vi "Grab images from pco.edge or pco.pixelfly CL test1.vi"() -> ()   [LabVIEW 2015]
doc: "A short program to demonstrate the fundamentals of control and image acquision with the pco.camera series. The program records a sequence of images, with \"live\" updating, until the \"StopRecording\" button is pressed. Use ctrl-H for more help on the individual controls and indicators.\n\nCopyright 2004, 2010 The Cooke Corporation."
panel:
  out "cam_fps":dbl=20.079713544692744 caption="FPS" format="%.1g"
  out "bClose":bool
  in  "Quit":bool
  out "BufNr1":i16
  out "BufNr0":i16
  in  "bUseBuffer1":bool
  in  "bUseBuffer0":bool
  in  "ROIX1":u16=1 min=1
  in  "ROIY1":u16=1 min=1
  in  "ROIY0":u16=1 min=1
  in  "ROIX0":u16=1 min=1
  out "Bits/pixel":u16
  in  "Record":bool
  in  "DelayTimeBase":u16(ring)=2 items=["nanoseconds", "microseconds", "milliseconds"]
  in  "ExposureTimeBase":u16(ring)=2 items=["nanoseconds", "microseconds", "milliseconds"]
  in  "Exposure":u32=10
  in  "Delay":u32
  in  "Rate":i32(ring) items=["95333333", "286000000"]
  out "Image":u16[][](graph)
  in  "TriggerMode":u16(ring) items=["Auto", "Software", "External sequence start ", "External exposure control"]
  # "A short program to demonstrate the fundamentals of control and image acquision with the pco.camera series. The program records a sequence of images, with \"live\" updating, until the \"StopRecording\" button is pressed.  Use ctrl-H for more help on the individual controls and indicators."
  # "pco.labview"
  # "1) Setup camera:"
  # "2) Record  images:"
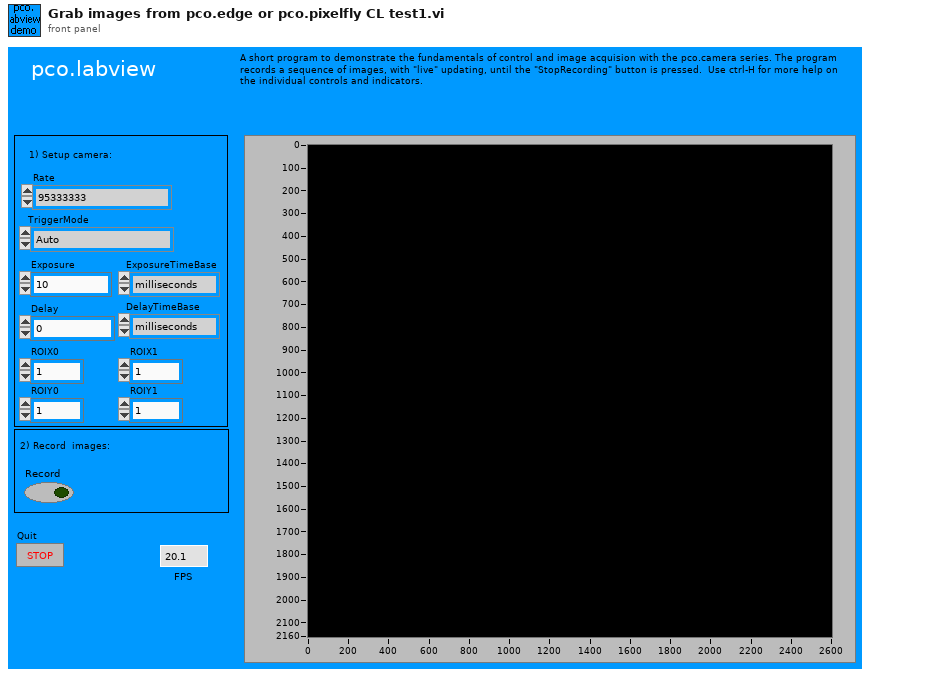
[diagram p1: front panel]
types:
  T1 = cluster{"SSize":u16, "CamType":u16, "CamsSubType":u16, "SerialNumber":u32, "HWVersion":u32, "FWVersion ":u32, "InterfaceType":u16, "HardwareVersions":cluster{"Board":u16, cluster{"string":string, "BatchNumber":u16, "MinorRevision":u8, "MajorRevision":u8, "Variant":u16}[]}, "FirmwareVersions":cluster{"DeviceNum":u16, cluster{"string":string, "MinorRevision":u8, "MajorRevision":u8, "Variant":u16}[]}}
  T2 = cluster{"Size":u16, "SensorTypeDESC":u16, "SensorSubtypeDESC":u16, "MaxHorizontalResStdDESC":u16, "MaxVerticalResStdDESC":u16, "MaxHorizontalResExtDESC":u16, "MaxVerticalResExtDESC":u16, "DynResDESC":u16, "MaxBinHorzDESC":u16, "BinHorzStepDESC":bool, "MaxBinVertDESC":u16, "BinVertStepDESC":bool, "ROIHorzStepDESC":u16, "ROIVertStepDESC":u16, "NumADCDESC":u16, "IRDESC":bool, "MinDelayDESC":u32, "MaxDelayDESC":u32, "MinDelayStepDESC":u32, "MinExpoDESC":u32, "MaxExpoDESC":u32, "MinExpoStepDESC":u32, "MinDelayIRDESC":u32, "MaxDelayIRDESC":u32, "MinExpoIRDESC":u32, "MaxExpoIRDESC":u32, "TimeTableDESC":bool, "DoubleImageDESC":bool, "MinCoolSetDESC":i16, "MaxCoolSetDESC":i16, "MDefaultCoolSetDESC":i16, "PowerDownModeDESC":bool, "OffsetRegDESC":bool, "ColorPattern":cluster{"UpperLeftColor":u8, "UpperRightColor":u8, "LowerLeftColor":u8, "LowerRightColor":u8}, "PatternTypeDESC":bool, "PixelRates":u32[], "CoversionFactors":u16[], "Reserved":u32[], "GeneralCapabilities":u32, "GeneralCapabilities 2":u32, "Min Size Hor":u16, "Min Size Vert":u16, "Ext Synch Freq":u32[], "Cooling Setpoints":i16[], "Soft ROI Hor Step":u16, "Soft ROI Vert Step":u16}
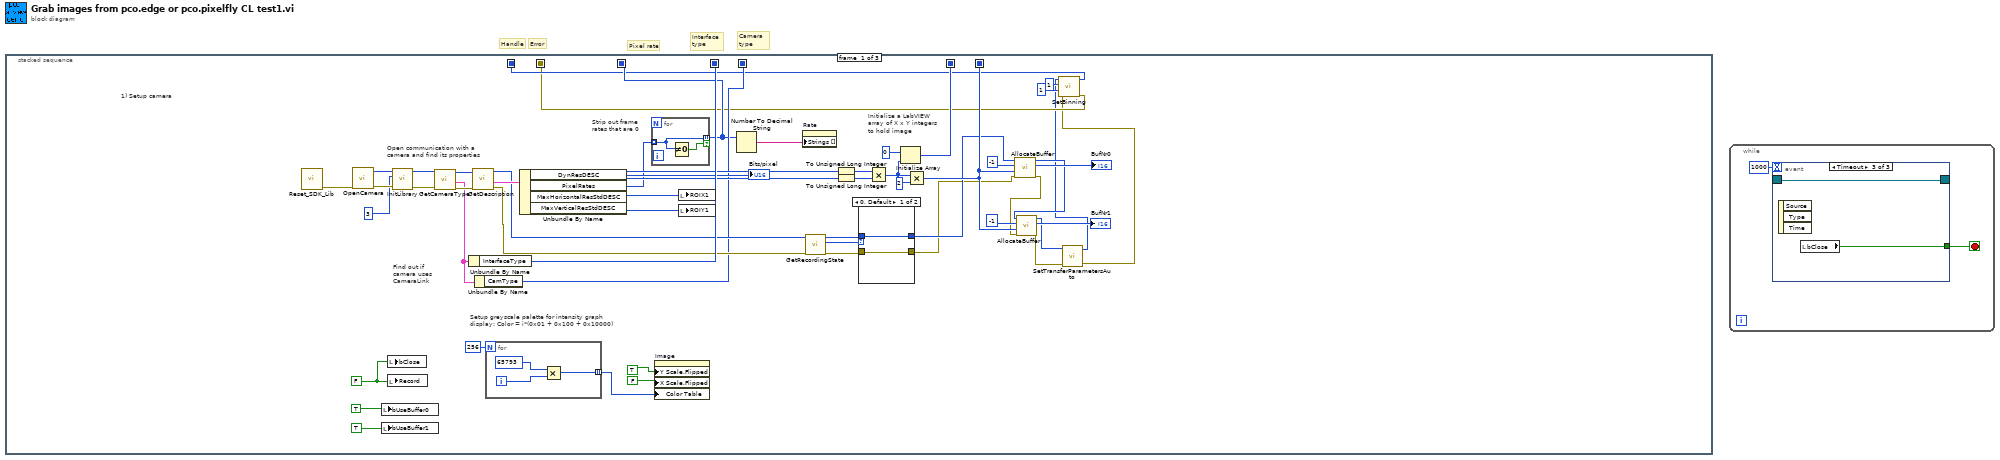
[diagram p0: block diagram]
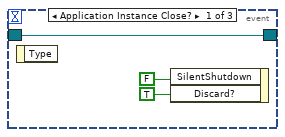
[diagram p2: hidden frame]
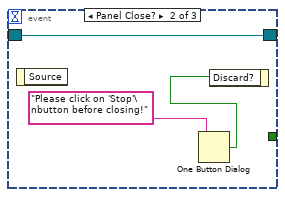
[diagram p3: hidden frame]
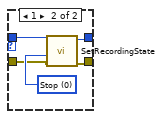
[diagram p4: hidden frame]
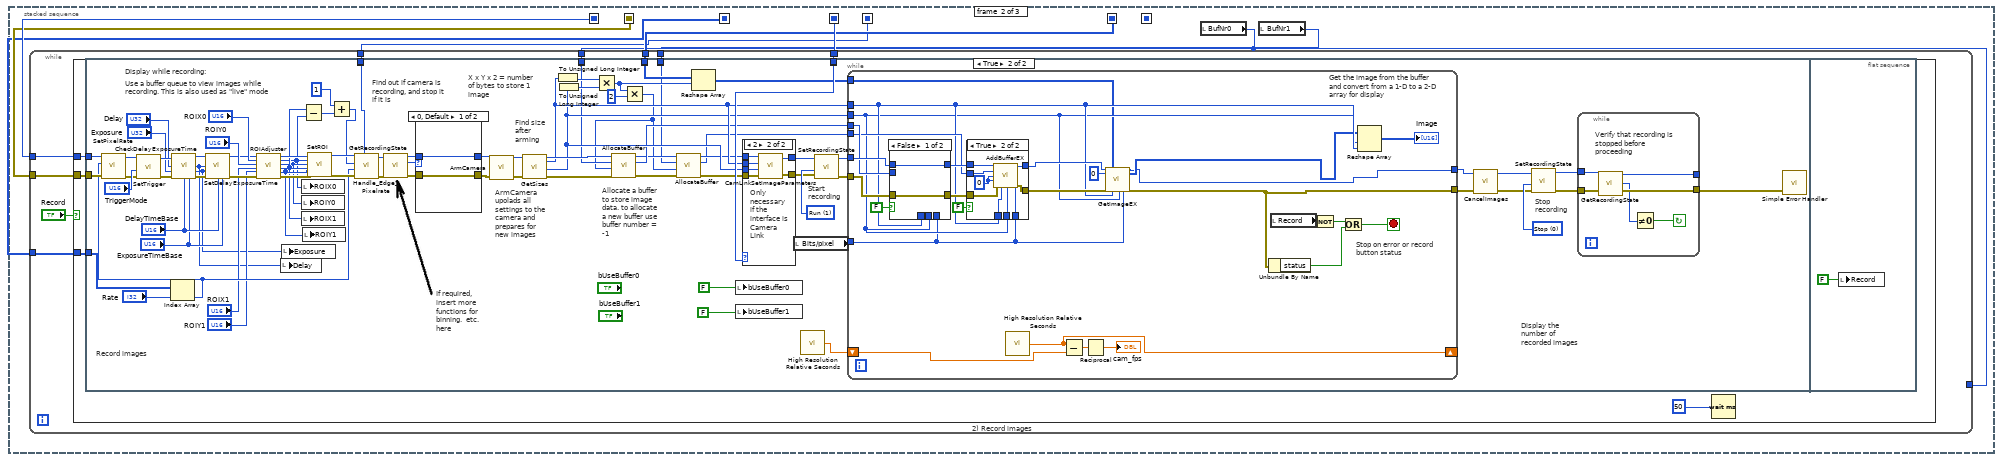
[diagram p5: hidden frame]
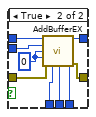
[diagram p7: hidden frame]
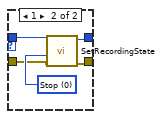
[diagram p10: hidden frame]
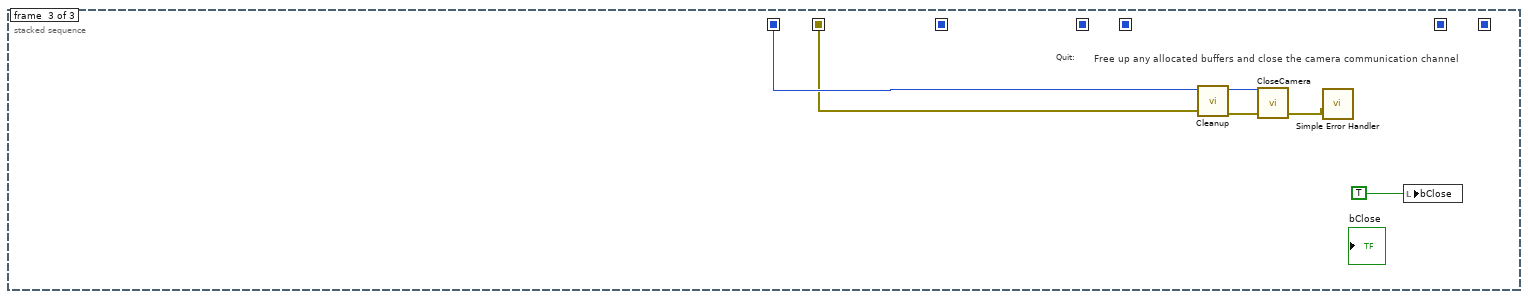
[diagram p11: hidden frame]
diagram:
  # "Camera type"
  # "Interface type"
  # "Error"
  # "Handle"
  # "Pixel rate"
  n1 = stacked-sequence {
    seq-local: [w47 _ _] -> [_ w70 _]
    seq-local: [w35 _ _] -> [_ _ _]
    seq-local: [w8 _ _] -> [_ w73 w247]
    seq-local: [w5 _ _] -> [_ w72 w246]
    seq-local: [w42 _ _] -> [_ w71 _]
    seq-local: [w9 _ _] -> [_ w67 _]
    seq-local: [w11 _ _] -> [_ w66 _]
    frame #0 {
      w29 = FALSE ("stop")
      # "Strip out frame rates that are 0"
      # "1) Setup camera"
      # "Find out if camera uses CameraLink"
      # "Setup greyscale palette for intensity graph display: Color = i*(0x01 + 0x100 + 0x10000)"
      # "Initialize a LabVIEW array of X x Y integers to hold image"
      # "Open communication with a camera and find its properties"
      n2 = call "Reset_SDK_Lib.vi"() -> ("ErrorOut"=w13:errorcluster)  [unwired: 11 in]
      n3 = call "OpenCamera.vi"("ErrorIn"=w13) -> ("ErrorOut"=w26:errorcluster, "Handle out"=w27:u64)  [unwired: 3 in, 2 out]
      n4 = local write "bUseBuffer0"(TRUE) -> ()
      n5 = local write "bUseBuffer1"(TRUE) -> ()
      n6 = local write "bClose"(w29) -> ()
      n7 = local write "Record"(w29) -> ()
      n8 = call "InitLibrary.vi"("error in (no error)"=w26, "InterfaceType"=u32 3, "ph"=w27) -> ("error out"=w25:errorcluster, "hout"=w24:u64)  [unwired: 7 in]
      n9 = call "GetCameraType.vi"("ph"=w24, "error in (no error)"=w25) -> ("hout"=w44:u64, "CameraType"=w12:T1, "error out"=w43:errorcluster)  [unwired: 1 in, 1 out]
      n10 = Unbundle By Name(w12) -> ("InterfaceType"=w42:u16)
      n11 = call "GetDescription.vi"("ErrorIn"=w43, "ph"=w44) -> ("ErrorOut"=w21:errorcluster, "Description"=w46:T2, "hout"=w20:u64)  [unwired: 2 in, 1 out]
      n12 = Unbundle By Name(w12) -> ("CamType"=w11:u16)
      n13 = for {
        N: 256 -> [_]
        tunnel: [w63] -> w50 mode=indexing
        i -> [w64]
        n14 = Multiply(x=65793, y=w64) -> (x*y=w63:i32)
      }
      n15 = Unbundle By Name(w46) -> ("DynResDESC"=→"Bits/pixel":u16, "PixelRates"=w10:u32[], "MaxHorizontalResStdDESC"=w40:u16, "MaxVerticalResStdDESC"=w39:u16)
      n16 = for {
        tunnel: w10 -> [w54] mode=indexing
        tunnel: [w54] -> w9 mode=indexing if=w55
        n17 = Not Equal To 0?(x=w54) -> (x != 0?=w55:bool)
      }
      n18 = property on="Image" class="IntGraph (strict)"("Y Scale.Flipped"=TRUE, "X Scale.Flipped"=FALSE, "Color Table"=w50) -> ()  [unwired: 2 in, 2 out]
      n19 = local write "ROIX1"(w40) -> ()
      n20 = local write "ROIY1"(w39) -> ()
      n21 = Number To Decimal String(number=w9) -> (decimal integer string=w28:string[])  [unwired: 1 in]
      n22 = property on="Rate" class="Ring (strict)"("Strings []"=w28) -> ()  [unwired: 2 in, 2 out]
      n23 = call "GetRecordingState.vi"("ErrorIn"=w21, "ph"=w20) -> ("ErrorOut"=w18:errorcluster, "Error"=w14:i32, "hout"=w19:u64)  [unwired: 2 in, 1 out]
      n24 = To Unsigned Long Integer(number=w40) -> (unsigned 32bit integer=w37:u32)
      n25 = To Unsigned Long Integer(number=w39) -> (unsigned 32bit integer=w36:u32)
      n26 = case shown="0, Default" w14 {
        tunnel: w19 -> [w57 w61]
        tunnel: w18 -> [w56 w60]
        tunnel: [w57 w59] -> w17
        tunnel: [w56 w58] -> w15
        frame 0, Default {
        }
        frame 1 {
          w62 = u16 0 items=["Stop", "Run"] ("RecordingState")
          n27 = call "SetRecordingState.vi"("ErrorIn"=w60, "RecordingState"=w62, "ph"=w61) -> ("ErrorOut"=w58:errorcluster, "hout"=w59:u64)  [unwired: 2 in, 1 out]
        }
      }
      n28 = Multiply(x=w37, y=w36) -> (x*y=w48:u32)
      n29 = Initialize Array(u16 0 ("Element Data"), w48) -> (w47:u16[])
      n30 = Multiply(x=w48, y=u32 2) -> (x*y=w35:u32)
      n31 = call "AllocateBuffer.vi"("error in (no error)"=w15, "Size"=w35, "BufNr"=i16 -1, "ph"=w17) -> ("error out"=w22:errorcluster, "BufNrOut"=→"BufNr0":i16, "hout"=w16:u64)  [unwired: 2 in, 3 out]
      n32 = call "AllocateBuffer.vi"("error in (no error)"=w22, "Size"=w35, "BufNr"=i16 -1, "ph"=w16) -> ("error out"=w2:errorcluster, "BufNrOut"=→"BufNr1":i16, "hout"=w4:u64)  [unwired: 2 in, 3 out]
      n33 = call "SetTransferParametersAuto.vi"("error in (no error)"=w2, "ph"=w4) -> ("error out"=w1:errorcluster, "hout"=w3:u64)  [unwired: 2 in, 1 out]
      n34 = call "SetBinning.vi"("error in (no error)"=w1, "BinVert"=u16 1, "BinHorz"=u16 1, "ph"=w3) -> ("error out"=w5:errorcluster, "hout"=w8:u64)  [unwired: 3 in, 1 out]
    }
    frame #1 {
      n35 = local read "BufNr0"() -> (w69:i16)
      n36 = local read "BufNr1"() -> (w68:i16)
      n37 = while {
        tunnel: w69 -> [_]
        tunnel: w69 -> [w79]
        tunnel: w70 -> [w81]
        tunnel: w71 -> [w82]
        tunnel: w72 -> [w80]
        tunnel: w73 -> [w77]
        tunnel: w68 -> [w78]
        tunnel: w67 -> [w75]
        tunnel: w66 -> [w74]
        stop <- "Quit" stop-if-true
        n38 = case "2) Record images" shown="True" "Record" {
          tunnel: w77 -> [_ w92]
          tunnel: w80 -> [_ w91]
          tunnel: w82 -> [_ w90]
          tunnel: w81 -> [_ w89]
          tunnel: w79 -> [_ w88]
          tunnel: w78 -> [_ w87]
          tunnel: w75 -> [_ w86]
          tunnel: w74 -> [_ w85]
          frame False {
          }
          frame True {
            n39 = flat-sequence {
              tunnel: w92 -> [w158]
              tunnel: w91 -> [w157]
              tunnel: w90 -> [w155]
              tunnel: w89 -> [w153]
              tunnel: w88 -> [w144]
              tunnel: w87 -> [w138]
              tunnel: w86 -> [w125]
              tunnel: w85 -> [w116]
              frame #0 {
                w171 = u16 1 items=["Stop", "Run"] ("RecordingState")
                w174 = u16 0 items=["Stop", "Run"] ("RecordingState")
                # "Display the number of recorded images"
                # "Record images"
                # "Start recording"
                # "Allocate a buffer to store image data. to allocate a new buffer use buffer number = -1"
                # "Find size after arming"
                # "ArmCamera upolads all settings to the camera and prepares for new images"
                # "Find out if camera is recording, and stop it if it is"
                # "If required, insert more functions for binning.  etc. here"
                # "X x Y x 2 = number of bytes to store 1 image"
                # "Stop recording"
                # "Use a buffer queue to view images while recording. This is also used as \"live\" mode"
                # "Display while recording:"
                n40 = Index Array(array=w125, index="Rate") -> (element=w120:u32)
                n41 = call "SetPixelRate.vi"("error in (no error)"=w157, "PixelRate"=w120, "ph"=w158) -> ("error out"=w127:errorcluster, "hout"=w128:u64)  [unwired: 2 in, 1 out]
                n42 = call "SetTrigger.vi"("error in (no error)"=w127, "TriggerMode"="TriggerMode", "ph"=w128) -> ("error out"=w101:errorcluster, "hout"=w103:u64)  [unwired: 2 in, 1 out]
                n43 = call "CheckDelayExposureTime.vi"("ph"=w103, "Delay"="Delay", "Exposure"="Exposure", "error in (no error)"=w101, "DelayTimeBase"="DelayTimeBase", "ExposureTimeBase"="ExposureTimeBase") -> ("hout"=w102:u64, "Delay Out"=w95:u32, "Exposure Out"=w94:u32, "error out"=w96:errorcluster)  [unwired: 4 in, 2 out]
                n44 = call "SetDelayExposureTime.vi"("ph"=w102, "Delay"=w95, "Exposure"=w94, "error in (no error)"=w96, "DelayTimeBase"="DelayTimeBase", "ExposureTimeBase"="ExposureTimeBase") -> ("hout"=w109:u64, "error out"=w115:errorcluster)  [unwired: 7 in, 1 out]
                n45 = call "ROIAdjuster.vi"("HandleIn"=w109, "ROIXmin"="ROIX0", "ROIYmin"="ROIY0", "ROIXmax"="ROIX1", "ROIYmax"="ROIY1", "ErrorIn"=w115) -> ("hout"=w108:u64, "ROIX0Mod"=w104:u16, "ROIY0Mod"=w105:u16, "ROIX1Mod"=w106:u16, "ROIY1Mod"=w107:u16, "ErrorOut"=w114:errorcluster)  [unwired: 7 in, 1 out]
                n46 = local write "Delay"(w95) -> ()
                n47 = local write "Exposure"(w94) -> ()
                n48 = Subtract(x=w106, y=w104) -> (x-y=w119:u16)
                n49 = local write "ROIX0"(w104) -> ()
                n50 = local write "ROIY0"(w105) -> ()
                n51 = local write "ROIX1"(w106) -> ()
                n52 = local write "ROIY1"(w107) -> ()
                n53 = call "SetROI.vi"("ph"=w108, "ROIX0"=w104, "ROIY0"=w105, "ROIX1"=w106, "ROIY1"=w107, "error in (no error)"=w114) -> ("hout"=w121:u64, "error out"=w122:errorcluster)  [unwired: 12 in]
                n54 = Add(x=1, y=w119) -> (x+y=w117:i32)
                n55 = call "Handle_Edge_Pixelrate.vi"("Cameratype"=w116, "error in (no error)"=w122, "PixelRate"=w120, "X-Resolution"=w117, "ph"=w121) -> ("error out"=w123:errorcluster, "hout"=w124:u64)  [unwired: 5 in]
                n56 = call "GetRecordingState.vi"("ErrorIn"=w123, "ph"=w124) -> ("ErrorOut"=w168:errorcluster, "RecordingState"=w170:u16, "hout"=w169:u64)  [unwired: 2 in, 1 out]
                n57 = case shown="0, Default" w170 {
                  tunnel: w169 -> [w239 w243]
                  tunnel: w168 -> [w238 w242]
                  tunnel: [w239 w241] -> w167
                  tunnel: [w238 w240] -> w166
                  frame 0, Default {
                  }
                  frame 1 {
                    w244 = u16 0 items=["Stop", "Run"] ("RecordingState")
                    n58 = call "SetRecordingState.vi"("ErrorIn"=w242, "RecordingState"=w244, "ph"=w243) -> ("ErrorOut"=w240:errorcluster, "hout"=w241:u64)  [unwired: 2 in, 1 out]
                  }
                }
                n59 = call "ArmCamera.vi"("error in (no error)"=w166, "ph"=w167) -> ("error out"=w164:errorcluster, "hout"=w165:u64)  [unwired: 1 in, 1 out]
                n60 = call "GetSizes.vi"("ph"=w165, "ErrorIn"=w164) -> ("hout"=w161:u64, "XResAct"=w151:u16, "YResAct"=w150:u16, "ErrorOut"=w163:errorcluster)  [unwired: 11 in, 3 out]
                n61 = To Unsigned Long Integer(number=w151) -> (unsigned 32bit integer=w145:u32)
                n62 = To Unsigned Long Integer(number=w150) -> (unsigned 32bit integer=w146:u32)
                n63 = Multiply(x=w145, y=w146) -> (x*y=w147:u32)
                n64 = Multiply(x=w147, y=u32 2) -> (x*y=w139:u32)
                n65 = call "AllocateBuffer.vi"("error in (no error)"=w163, "Size"=w139, "BufNr"=w144, "ph"=w161) -> ("error out"=w143:errorcluster, "BufNrOut"=w148:i16, "hout"=w141:u64)  [unwired: 2 in, 3 out]
                n66 = call "AllocateBuffer.vi"("error in (no error)"=w143, "Size"=w139, "BufNr"=w138, "ph"=w141) -> ("error out"=w142:errorcluster, "BufNrOut"=w137:i16, "hout"=w140:u64)  [unwired: 2 in, 3 out]
                n67 = Reshape Array(w153, w147) -> (w152:u16[])
                n68 = local write "bUseBuffer0"(FALSE) -> ()
                n69 = local write "bUseBuffer1"(FALSE) -> ()
                n70 = case shown="2" w155 {
                  tunnel: w142 -> [w230 w237]
                  tunnel: [w230 w236] -> w160
                  tunnel: w140 -> [w231 w235]
                  tunnel: [w231 w234] -> w159
                  tunnel: w150 -> [_ w233]
                  tunnel: w151 -> [_ w232]
                  frame 0, Default {
                  }
                  frame 2 {
                    # "Only necessary if the interface is Camera Link"
                    n71 = call "CamLinkSetImageParameters.vi"("error in (no error)"=w237, "YRes"=w233, "XRes"=w232, "ph"=w235) -> ("error out"=w236:errorcluster, "hout"=w234:u64)  [unwired: 1 out]
                  }
                }
                n72 = local read "Bits/pixel"() -> (w132:u16)
                n73 = call <vilib>:"High Resolution Relative Seconds.vi"() -> ("relative seconds"=w93:dbl)
                n74 = call "SetRecordingState.vi"("ErrorIn"=w160, "RecordingState"=w171, "ph"=w159) -> ("ErrorOut"=w156:errorcluster, "hout"=w154:u64)  [unwired: 2 in, 1 out]
                n75 = while {
                  tunnel: w148 -> [w195]
                  tunnel: w152 -> [w177]
                  tunnel: w154 -> [w200]
                  tunnel: w150 -> [w182]
                  tunnel: w151 -> [w183]
                  tunnel: w156 -> [w198]
                  tunnel: [w179] -> w131
                  tunnel: [w178] -> w130
                  tunnel: w137 -> [w194]
                  tunnel: w132 -> [w181]
                  shift-right: [w187] -> _
                  shift-left: w93 -> [w188]
                  stop <- w191 stop-if-true
                  # "Stop on error or record button status"
                  # "Get the image from the buffer and convert from a 1-D to a 2-D array for display"
                  n76 = case shown="False" FALSE {
                    tunnel: [w203 w212] -> w197
                    tunnel: [w202 w211] -> w199
                    tunnel: w195 -> [_ w210]
                    tunnel: w200 -> [w202 w209]
                    tunnel: w181 -> [_ w207]
                    tunnel: w183 -> [_ w206]
                    tunnel: w182 -> [_ w205]
                    tunnel: w198 -> [w203 w204]
                    frame False {
                    }
                    frame True {
                      w208 = i16 0
                      n77 = call "AddBufferEX.vi"("ph"=w209, "BuffNr"=w210, "1stImage"=w208, "LastImage"=w208, "error in (no error)"=w204, "XRes"=w206, "YRes"=w205, "BitPerPixel"=w207) -> ("hout"=w211:u64, "error out"=w212:errorcluster)  [unwired: 5 in, 1 out]
                    }
                  }
                  n78 = case shown="True" FALSE {
                    tunnel: [w213 w223] -> w186
                    tunnel: [w214 w222] -> w184
                    tunnel: w194 -> [_ w221]
                    tunnel: w199 -> [w214 w220]
                    tunnel: w181 -> [_ w218]
                    tunnel: w183 -> [_ w217]
                    tunnel: w182 -> [_ w216]
                    tunnel: w197 -> [w213 w215]
                    frame False {
                    }
                    frame True {
                      w219 = i16 0
                      n79 = call "AddBufferEX.vi"("ph"=w220, "BuffNr"=w221, "1stImage"=w219, "LastImage"=w219, "error in (no error)"=w215, "XRes"=w217, "YRes"=w216, "BitPerPixel"=w218) -> ("hout"=w222:u64, "error out"=w223:errorcluster)  [unwired: 5 in, 1 out]
                    }
                  }
                  n80 = call <vilib>:"High Resolution Relative Seconds.vi"() -> ("relative seconds"=w187:dbl)
                  n81 = Subtract(x=w187, y=w188) -> (x-y=w190:dbl)
                  n82 = Reciprocal(x=w190) -> (1/x=→"cam_fps":dbl)
                  n83 = call "GetImageEX.vi"("ph"=w184, "BuffNr"=i16 0, "error in (no error)"=w186, "BuffIn"=w177, "xRes"=w183, "yRes"=w182, "BitPerPixel"=w181) -> ("hout"=w179:u64, "BuffOut"=w180:u16[], "error out"=w178:errorcluster)  [unwired: 9 in, 1 out]
                  n84 = Unbundle By Name(w178) -> ("status"=w192:bool)
                  n85 = local read "Record"() -> (w201:bool)
                  n86 = Not(x=w201) -> (.not. x?=w193:bool)
                  n87 = Or(x=w193, y=w192) -> (x .or. y?=w191:bool)
                  n88 = Reshape Array(w180, w182, w183) -> (→"Image":u16[][])
                }
                n89 = call "CancelImages.vi"("error in (no error)"=w130, "ph"=w131) -> ("error out"=w134:errorcluster, "hout"=w133:u64)  [unwired: 1 in, 1 out]
                n90 = call "SetRecordingState.vi"("ErrorIn"=w134, "RecordingState"=w174, "ph"=w133) -> ("ErrorOut"=w172:errorcluster, "hout"=w173:u64)  [unwired: 2 in, 1 out]
                n91 = while {
                  tunnel: [w227] -> w129
                  tunnel: w172 -> [w228]
                  tunnel: w173 -> [w229]
                  tunnel: [w224] -> _
                  stop <- w225 continue-if-true
                  # "Verify that recording is stopped before proceeding"
                  n92 = call "GetRecordingState.vi"("ErrorIn"=w228, "ph"=w229) -> ("ErrorOut"=w227:errorcluster, "RecordingState"=w226:u16, "hout"=w224:u64)  [unwired: 2 in, 1 out]
                  n93 = Not Equal To 0?(x=w226) -> (x != 0?=w225:bool)
                }
                n94 = call <vilib>:"Simple Error Handler.vi"("error in (no error)"=w129) -> ()  [unwired: 4 in, 5 out]
              }
              frame #1 {
                n95 = local write "Record"(FALSE ("Record")) -> ()
              }
            }
          }
        }
        n96 = Wait (ms)(milliseconds to wait=u32 50) -> ()  [unwired: 1 out]
      }
    }
    frame #2 {
      # "Free up any allocated buffers and close the camera communication channel"
      # "Quit:"
      n97 = call "Cleanup.vi"("error in (no error)"=w246, "ph"=w247) -> ("error out"=w248:errorcluster, "hout"=w249:u64)  [unwired: 8 in]
      n98 = call "CloseCamera.vi"("ErrorIn"=w248, "Handle in"=w249) -> ("ErrorOut"=w251:errorcluster)  [unwired: 1 in, 2 out]
      n99 = call <vilib>:"Simple Error Handler.vi"("error in (no error)"=w251) -> ()  [unwired: 4 in, 5 out]
      n100 = local write "bClose"(TRUE) -> ()
    }
  }
  n101 = while {
    stop <- w252 stop-if-true
    n102 = event shown="[2] Timeout" {
      selector: _ -> [w254 w259 w261]
      dyn-events: [w254 w259 w261] -> _
      timeout: 1000 -> [_ _ _]
      tunnel: [_ _ w260] -> w252
      event Application Instance Close? {
        n103 = event-data() -> ()  [unwired: 1 in, 1 out]
        n104 = event-data("SilentShutdown"=FALSE, "Discard?"=TRUE) -> ()  [unwired: 1 in, 1 out]
      }
      event Panel Close? {
        n105 = event-data() -> ()  [unwired: 1 in, 1 out]
        n106 = One Button Dialog(message="Please click on 'Stop'\nbutton before closing!") -> (true=w257:bool)  [unwired: 1 in]
        n107 = event-data("Discard?"=w257) -> ()  [unwired: 1 in, 1 out]
      }
      event Timeout {
        n108 = event-data() -> ()  [unwired: 1 in, 3 out]
        n109 = local read "bClose"() -> (w260:bool)
      }
    }
  }
